vi "PH_Beckhoff_StepMot.declare analog OutputTags.vi"(3 "Instance Name":string="N/A") -> (0 "Analog Outputs":T1, 1 "Description":string)   [LabVIEW 2014, in "PH_Beckhoff_StepMot.lvlib"]
uses:
  PH_Beckhoff_StepMot.lvlib
  PH_Beckhoff/PH_Beckhoff.Analog Outputs.ctl
  PH_Beckhoff/PH_Beckhoff.Scaling Type.ctl
  PH_Beckhoff/PH_Beckhoff.lvlib
panel:
  out "Right Size?":bool
  # "Let this VI run to check the size!"
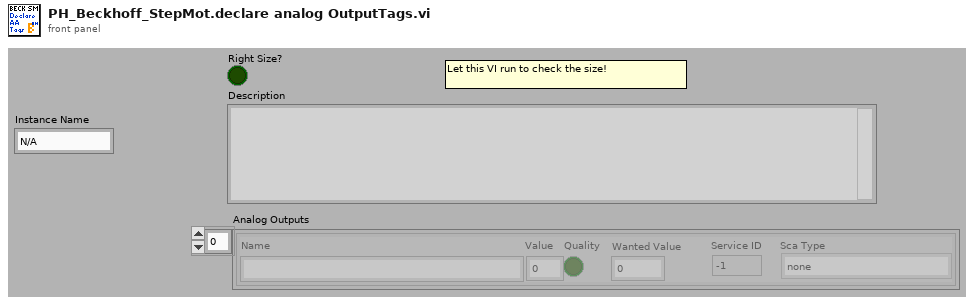
[diagram p1: front panel]
types:
  T1 = typedef "PH_Beckhoff.lvlib/PH_Beckhoff.Analog Outputs.ctl" = cluster{"Name":string, "Value":u32, "Quality":bool, "Wanted Value":u32, "Service ID":i32, "Sca Type":T2}[]
  T2 = typedef "PH_Beckhoff.lvlib/PH_Beckhoff.Scaling Type.ctl" = enum16{"none", "0 ... 15 Bit -> 0 ... 5", "0 ... 15 Bit -> 0 ... 10", "0 ... 15 Bit -> 0 ... 25", "0 ... 15 Bit -> 4 ... 20", "0 ... 15 Bit -> 0 ... 1", "0 ... 15 Bit -> 0 ... 20000", "0 ... 15 Bit -> 0 ... 24000"}
  T3 = cluster{"Name":string, "Value":u32, "Quality":bool, "Wanted Value":u32, "Service ID":i32, "Sca Type":T2}
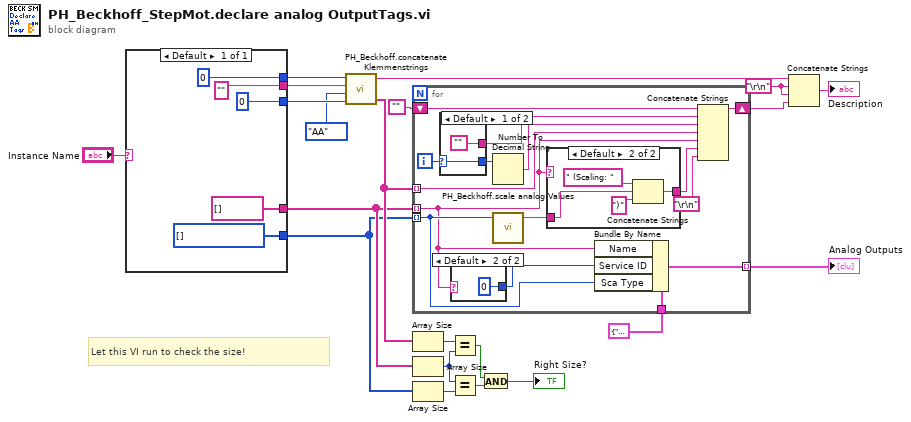
[diagram p0: block diagram]
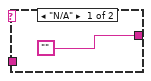
[diagram p2: hidden frame]
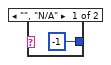
[diagram p3: hidden frame]
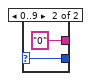
[diagram p4: hidden frame]
diagram:
  w19 = "\r\n"
  # "Let this VI run to check the size!"
  n1 = case shown="Default" "Instance Name" {
    tunnel: ["" ("Klemmenname")] -> w15
    tunnel: [0 ("# of In- or Outputs")] -> w14
    tunnel: [0 ("Quantity")] -> w9
    tunnel: [string[] []] -> w3
    tunnel: [w22] -> w2
    frame Default {
      w22 = T2[] [] items=["none", "0 ... 15 Bit -> 0 ... 5", "0 ... 15 Bit -> 0 ... 10", "0 ... 15 Bit -> 0 ... 25", "0 ... 15 Bit -> 4 ... 20", "0 ... 15 Bit -> 0 ... 1", "0 ... 15 Bit -> 0 ... 20000", "0 ... 15 Bit -> 0 ... 24000"]
    }
  }
  n2 = call "PH_Beckhoff.concatenate Klemmenstrings.vi"("# of In- or Outputs"=w14, "Type"=enum16{"AE", "AA", "DE", "DA", "SE"}."AA", "Klemmenname"=w15, "Quantity"=w9) -> ("concatenated string array"=w7:string[], "\"<Type>: <Quantity> x <Klemmenname>\""=w8:string)  [unwired: 1 out]
  n3 = for {
    tunnel: w3 -> [w27] mode=indexing
    tunnel: w7 -> [w37] mode=indexing
    shift-right: [w29] -> w20
    shift-left: "" -> [w30]
    tunnel: w2 -> [w33] mode=indexing
    tunnel: T3 {"Name"="", "Value"=0, "Quality"=FALSE, "Wanted Value"=0, "Service ID"=0, "Sca Type"=enum."none"} ("Analog Output Value") -> [w32]
    tunnel: [w34] -> w5 mode=indexing
    i -> [w41]
    n4 = case shown="Default" w41 {
      selector: w41 -> [w49 w52]
      tunnel: [w49 w52] -> w40
      tunnel: ["" "0"] -> w39
      frame Default {
      }
      frame 0..9 {
      }
    }
    n5 = case shown="Default" w27 {
      tunnel: [-1 ("Service ID") 0 ("Service ID")] -> w35
      frame "", "N/A" {
      }
      frame Default {
      }
    }
    n6 = Number To Decimal String(number=w40) -> (decimal integer string=w38:string)  [unwired: 1 in]
    n7 = call "PH_Beckhoff.scale analog Values.vi"("Sca Type"=w33) -> ("Scaling"=w31:string)  [unwired: 2 in, 2 out]
    n8 = case shown="Default" w27 {
      tunnel: ["" w45] -> w36
      tunnel: w31 -> [_ w44]
      frame "N/A" {
      }
      frame Default {
        n9 = Concatenate Strings(" (Scaling: " ("string"), w44, ")" ("string")) -> (w45:string)
      }
    }
    n10 = Bundle By Name(cluster=w32, "Name"=w27, "Service ID"=w35, "Sca Type"=w33) -> (w34:T3)
    n11 = Concatenate Strings(w30, w39, w38, w37, w27, w36, "\r\n") -> (w29:string)
  }
  "Analog Outputs" <- w5
  n12 = Array Size(array=w7) -> (size(s)=w17:i32)
  n13 = Array Size(array=w3) -> (size(s)=w13:i32)
  n14 = Array Size(array=w2) -> (size(s)=w12:i32)
  n15 = Equal?(x=w17, y=w13) -> (x = y?=w16:bool)
  n16 = Equal?(x=w13, y=w12) -> (x = y?=w10:bool)
  n17 = And(x=w16, y=w10) -> (x .and. y?=→"Right Size?":bool)
  n18 = Concatenate Strings(w8, w19, w19, w20) -> (→"Description":string)
